vi "EIP Sub Channel.vi"(8 "error in (no error)":errorcluster, 11 "Node Ptr":T2 format="%.0x") -> (0 "error out":errorcluster)   [LabVIEW 2023, in "Ethernet IP Custom Device Custom Device.lvlib"]
uses:
  <vilib>/NI VeriStand/Custom Device API/Custom Device Item Ref.ctl
  L5K Data Types.ctl
  Ethernet IP Global Strings.vi
  <vilib>/NI VeriStand/Custom Device API/Get Item Property (String).vi
  <vilib>/NI VeriStand/Custom Device API/Get Item Property (U16).vi
  Ethernet IP Custom Device Custom Device.lvlib
  <vilib>/NI VeriStand/Custom Device API/Custom Device API.lvlib
panel:
  in  "Default Value":dbl
  out "Data Type":T1
  in  "Description":string
  out "Tag Name":string
  in  "Header":cluster{"Section Name":string}={"Section Name"="Custom Device Item Settings"}
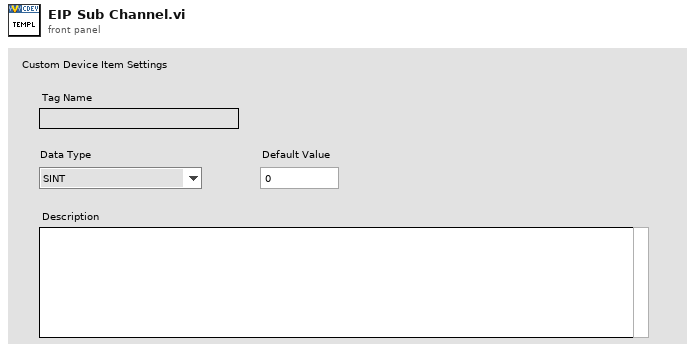
[diagram p1: front panel]
types:
  T1 = typedef "Ethernet IP Custom Device Custom Device.lvlib/L5K Data Types.ctl" = enum16{"SINT", "INT", "DINT", "REAL", "BOOL"}
  T2 = typedef "Custom Device API.lvlib/Custom Device Item Ref.ctl" = u64
  T3 = typedef "Custom Device API.lvlib/Custom Device Channel.ctl" = cluster{"Type":T4, "Units":string, "Default Value":dbl, "Faultable":bool, "Scalable":bool}
  T4 = typedef "Custom Device API.lvlib/Custom Device Channel Type.ctl" = enum16{"Input", "Output"}
  T5 = typedef "Custom Device API.lvlib/Custom Device Commands.ctl" = enum16{"Default", "Item renamed", "Shutdown", "Dynamic button pressed"}
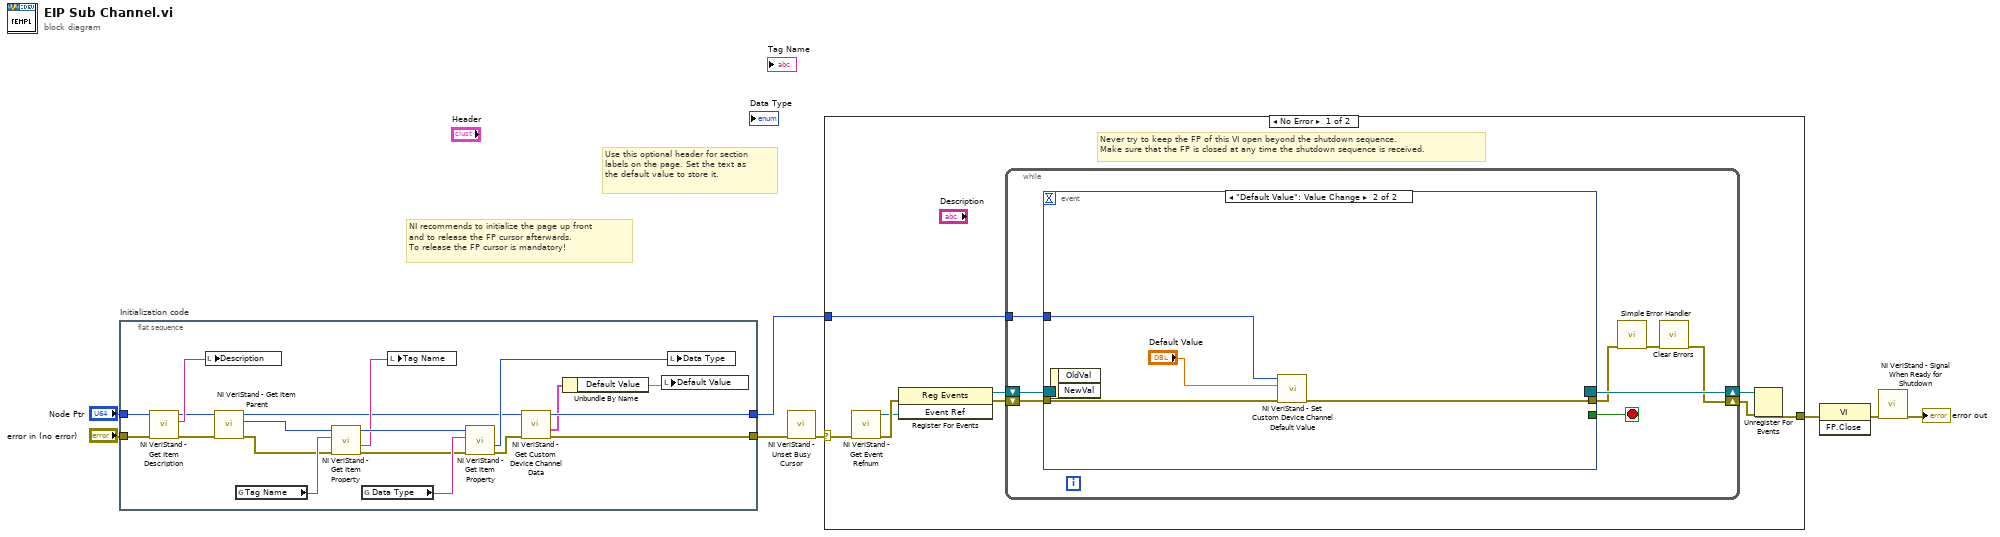
[diagram p0: block diagram]
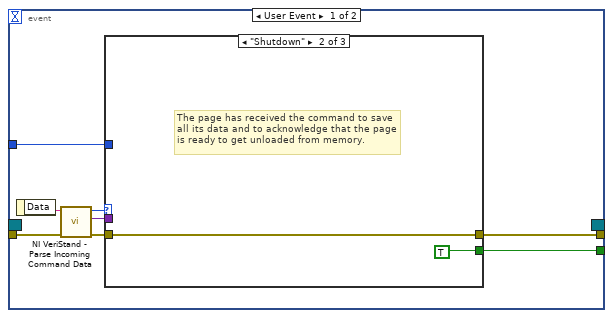
[diagram p2: hidden frame]
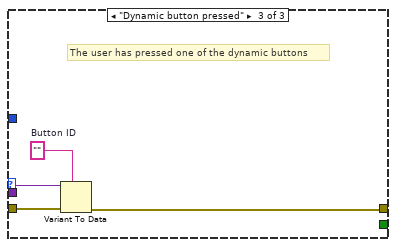
[diagram p4: hidden frame]
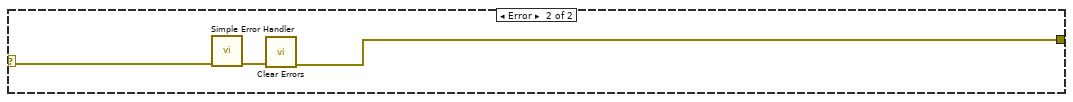
[diagram p5: hidden frame]
diagram:
  # "Use this optional header for section labels on the page. Set the text as the default value to store it."
  # "NI recommends to initialize the page up front\nand to release the FP cursor afterwards.\nTo release the FP cursor is mandatory!"
  n1 = flat-sequence "Initialization code" {
    tunnel: "error in (no error)" -> [w27]
    tunnel: "Node Ptr" -> [w26]
    tunnel: [w13] -> w2
    tunnel: [w11] -> w1
    frame #0 {
      n2 = call <vilib>:"NI VeriStand - Get Item Description.vi"("error in (no error)"=w27, "Item Ref in"=w26) -> ("error out"=w24:errorcluster, "Description"=w25:string, "Item Ref out"=w23:T2)  [unwired: 7 out]
      n3 = local write "Description"(w25) -> ()
      n4 = call <vilib>:"NI VeriStand - Get Item Parent.vi"("error in (no error)"=w24, "Item Ref in"=w23) -> ("error out"=w17:errorcluster, "Parent Ref"=w18:T2, "Item Ref out"=w14:T2)  [unwired: 6 in, 1 out]
      n5 = global read "Ethernet IP Global Strings.vi" "Tag Name"() -> (w22:string)
      n6 = call-poly <vilib>:"NI VeriStand - Get Item Property.vi"("error in (no error)"=w17, "Property Name"=w22, "Item Ref in"=w18) -> ("error out"=w19:errorcluster, "Value"=w16:string, "Item Ref out"=w20:T2)  [unwired: 5 in, 1 out]
      n7 = global read "Ethernet IP Global Strings.vi" "Data Type"() -> (w21:string)
      n8 = local write "Tag Name"(w16) -> ()
      n9 = call-poly <vilib>:"NI VeriStand - Get Item Property.vi"("error in (no error)"=w19, "Property Name"=w21, "Item Ref in"=w20) -> ("error out"=w12:errorcluster, "Value"=w15:u16)  [unwired: 5 in, 2 out]
      n10 = call <vilib>:"NI VeriStand - Get Custom Device Channel Data.vi"("error in (no error)"=w12, "Channel Ref in"=w14) -> ("error out"=w11:errorcluster, "Channel"=w10:T3, "Channel Ref out"=w13:T2)  [unwired: 4 in, 3 out]
      n11 = Unbundle By Name(w10) -> ("Default Value"=w9:dbl)
      n12 = local write "Default Value"(w9) -> ()
      n13 = local write "Data Type"(w15) -> ()
    }
  }
  n14 = call <vilib>:"NI VeriStand - Unset Busy Cursor.vi"("error in (no error)"=w1) -> ("error out"=w4:errorcluster)  [unwired: 10 out]
  n15 = case shown="No Error" w4 {
    selector: w4 -> [w28 w66]
    tunnel: [w33 w64] -> w8
    tunnel: w2 -> [w29 _]
    frame No Error {
      # "Never try to keep the FP of this VI open beyond the shutdown sequence.\nMake sure that the FP is closed at any time the shutdown sequence is received."
      n16 = call <vilib>:"NI VeriStand - Get Event Refnum.vi"("error in (no error)"=w28) -> ("error out"=w36:errorcluster, "Event Ref"=w32:refnum<user-event>)  [unwired: 9 out]
      n17 = register-events(error in=w36, w32) -> (reference out=w30:refnum<event-registration>, error out=w31:errorcluster)  [unwired: 1 in]
      n18 = while {
        tunnel: w29 -> [w40]
        shift-right: [w37] -> w34
        shift-left: w31 -> [w43]
        shift-right: [w44] -> w35
        shift-left: w30 -> [w42]
        stop <- w41 stop-if-true
        n19 = event shown="[1] \"Default Value\": Value Change" {
          selector: w42 -> [_ _]
          dyn-events: [_ _] -> w44
          timeout: _ -> [_ _]
          tunnel: w43 -> [w52 w63]
          tunnel: [w48 _] -> w41
          tunnel: [w47 w60] -> w39
          tunnel: w40 -> [w46 w62]
          event User Event {
            n20 = event-data() -> ("Data"=w51:string)  [unwired: 1 out]
            n21 = call <vilib>:"NI VeriStand - Parse Incoming Command Data.vi"("error in (no error)"=w52, "Incoming data"=w51) -> ("error out"=w50:errorcluster, "Outgoing data"=w45:variant, "Action"=w49:T5)  [unwired: 7 out]
            n22 = case shown="\"Shutdown\"" w49 {
              tunnel: w50 -> [w53 w54 w59]
              tunnel: [_ TRUE _] -> w48
              tunnel: [w53 w54 w56] -> w47
              tunnel: w46 -> [_ _ _]
              tunnel: w45 -> [_ _ w58]
              frame "Default", Default {
              }
              frame "Shutdown" {
                # "The page has received the command to save all its data and to acknowledge that the page is ready to get unloaded from memory."
              }
              frame "Dynamic button pressed" {
                w57 = ""  # Button ID
                # "The user has pressed one of the dynamic buttons"
                n23 = Variant To Data(error in=w59, type=w57, Variant=w58) -> (error out=w56:errorcluster)  [unwired: 1 out]
              }
            }
          }
          event "Default Value": Value Change {
            n24 = event-data() -> ()  [unwired: 3 out]
            n25 = call <vilib>:"NI VeriStand - Set Custom Device Channel Default Value.vi"("error in (no error)"=w63, "Default Value"="Default Value", "Channel Ref in"=w62) -> ("error out"=w60:errorcluster)  [unwired: 7 in, 1 out]
          }
        }
        n26 = call <vilib>:"Simple Error Handler.vi"("error in (no error)"=w39) -> ("error out"=w38:errorcluster)  [unwired: 1 in, 7 out]
        n27 = call <vilib>:"Clear Errors.vi"("error in (no error)"=w38) -> ("error out"=w37:errorcluster)  [unwired: 1 in, 5 out]
      }
      n28 = Unregister For Events(event registration refnum=w35, error in=w34) -> (error out=w33:errorcluster)
    }
    frame Error {
      n29 = call <vilib>:"Simple Error Handler.vi"("error in (no error)"=w66) -> ("error out"=w65:errorcluster)  [unwired: 1 in, 7 out]
      n30 = call <vilib>:"Clear Errors.vi"("error in (no error)"=w65) -> ("error out"=w64:errorcluster)  [unwired: 1 in, 5 out]
    }
  }
  n31 = invoke class="VI" method="FP.Close"(error in=w8) -> (error out=w7:errorcluster)  [unwired: 2 in, 2 out]
  n32 = call <vilib>:"NI VeriStand - Signal When Ready for Shutdown.vi"("error in (no error)"=w7) -> ("error out"=→"error out":errorcluster)  [unwired: 10 out]
